vi "pf_Extract_Camera_Properties.vi"(8 "error in (no error)":errorcluster, 11 "IMAQ Session in":refnum<k11>) -> (0 "error out":errorcluster, 1 "Properties Array":T1[](array[typedef]), 3 "IMAQ Session out":refnum<k11>)   [LabVIEW 2025, in "Photonfocus_Toolkit.lvlib"]
uses:
  Photonfocus_Toolkit.lvlib
  _Private/Controls/pf_Property_Cluster.ctl
  _Private/Controls/pf_Property_Type.ctl
  _Private/Controls/pf_Property_Flag.ctl
  _Private/Controls/pf_Property_Info.ctl
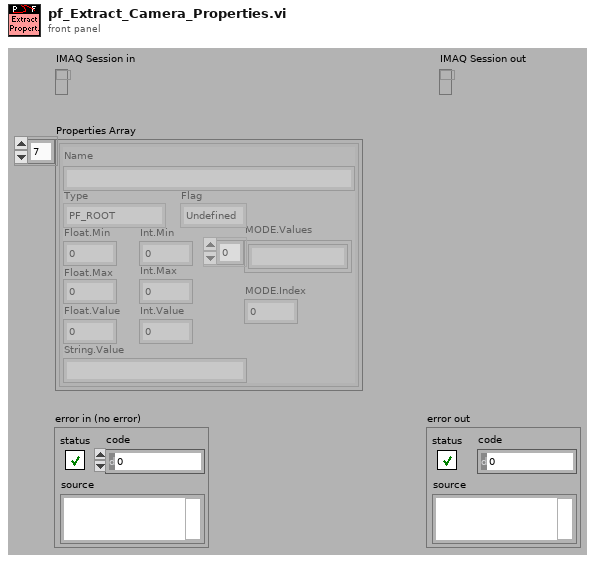
[diagram p1: front panel]
types:
  T1 = typedef "Photonfocus_Toolkit.lvlib/pf_Property_Cluster.ctl" = cluster{"Name":string, "Type":T2, "Float.Min":sgl, "Float.Max":sgl, "Float.Value":sgl, "Int.Min":u32, "Int.Max":u32, "Int.Value":u32, "String.Value":string, "MODE.Values":string[], "MODE.Index":i32, "Flag":T3}
  T2 = typedef "Photonfocus_Toolkit.lvlib/pf_Property_Type.ctl" = enum16{"Undefined", "PF_ROOT", "PF_INT", "PF_FLOAT", "PF_BOOL", "PF_MODE", "PF_REGISTER", "PF_STRING", "PF_BUFFER", "PF_STRUCT", "PF_ARRAY", "PF_COMMAND", "PF_EVENT"}
  T3 = typedef "Photonfocus_Toolkit.lvlib/pf_Property_Flag.ctl" = enum16{"Undefined", "RO", "WO", "RW"}
  T4 = typedef "Photonfocus_Toolkit.lvlib/pf_Property_Info.ctl" = cluster{"Name":string, "Type":T2, "Flag":T3}
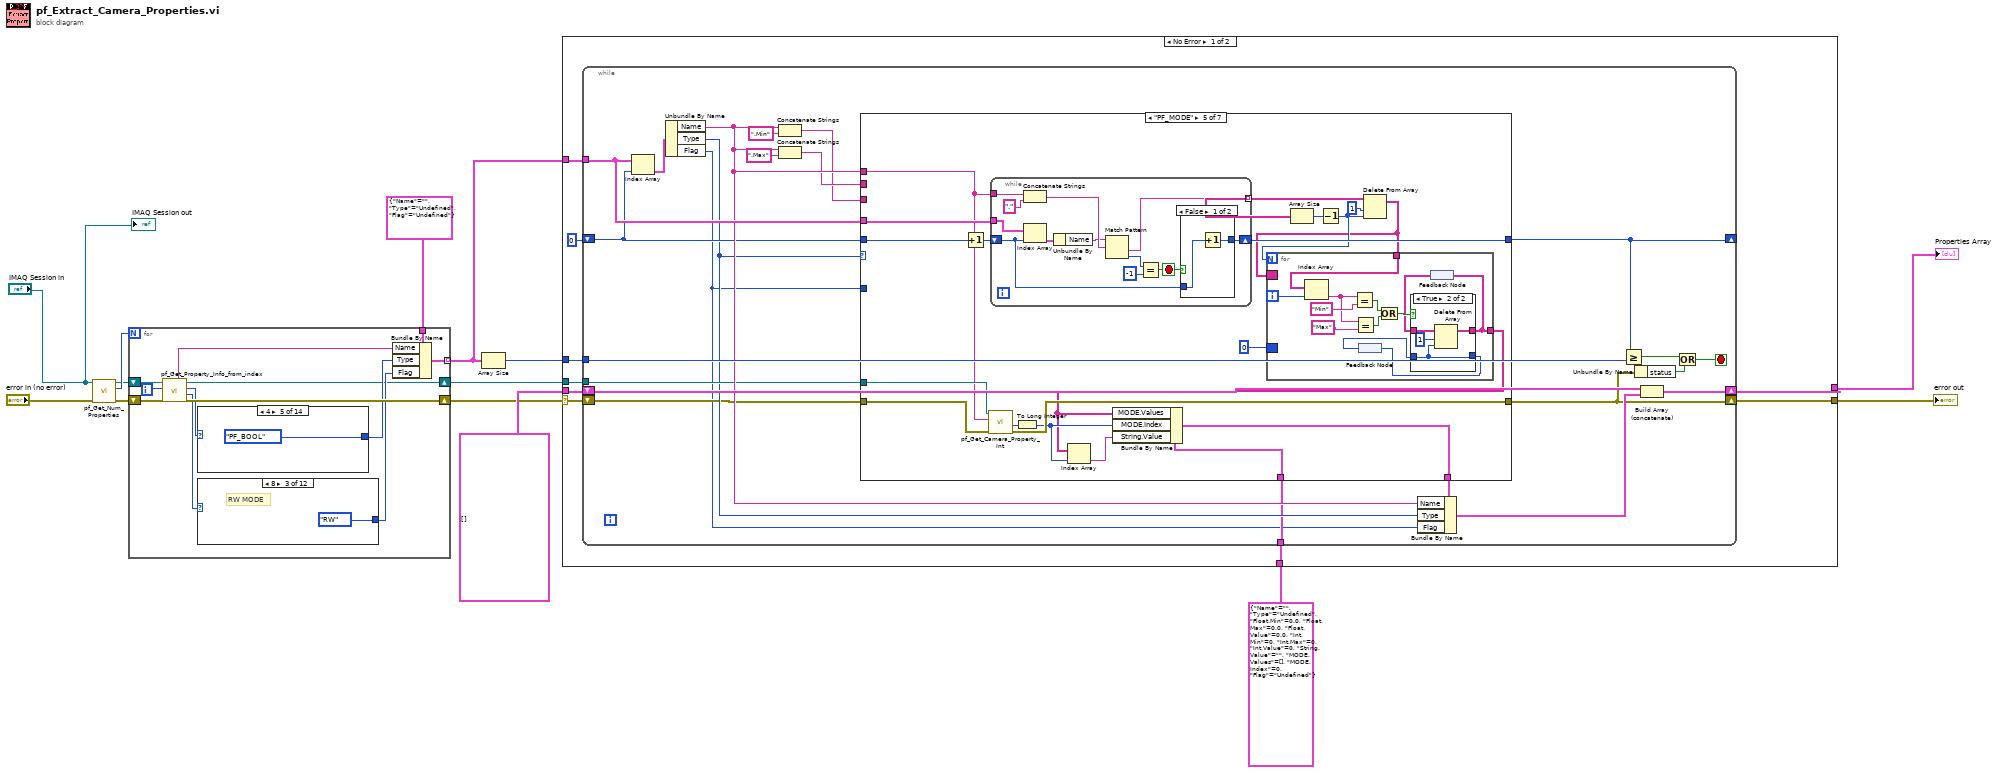
[diagram p0: block diagram]
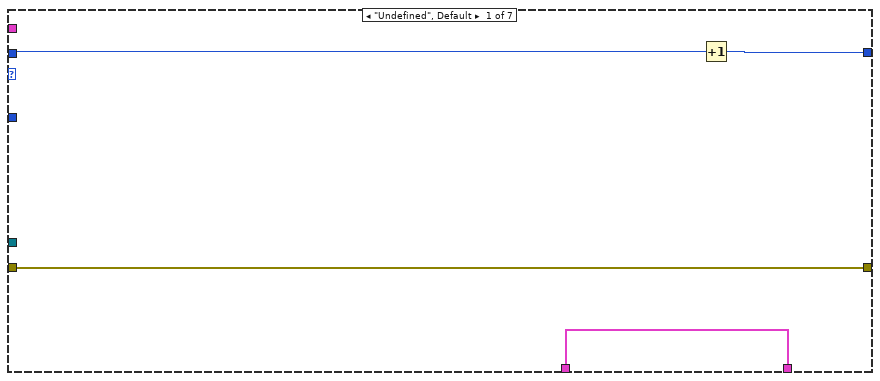
[diagram p2: hidden frame]
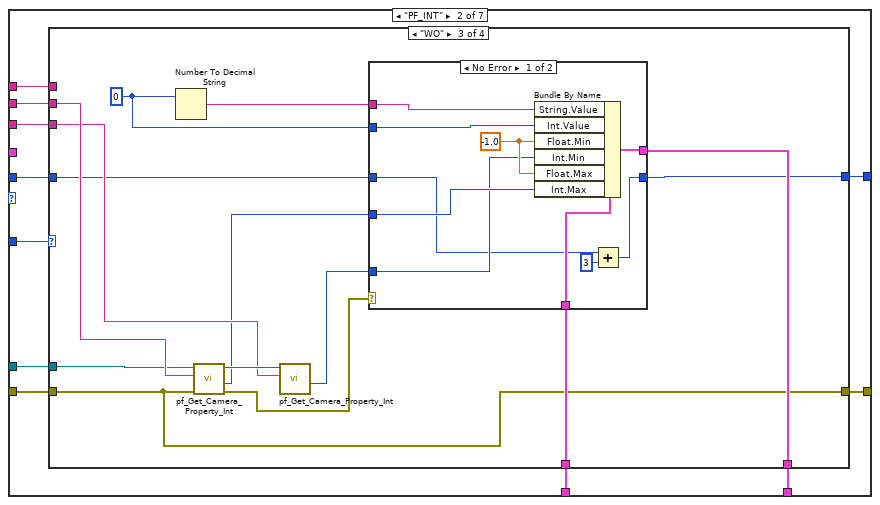
[diagram p3: hidden frame]
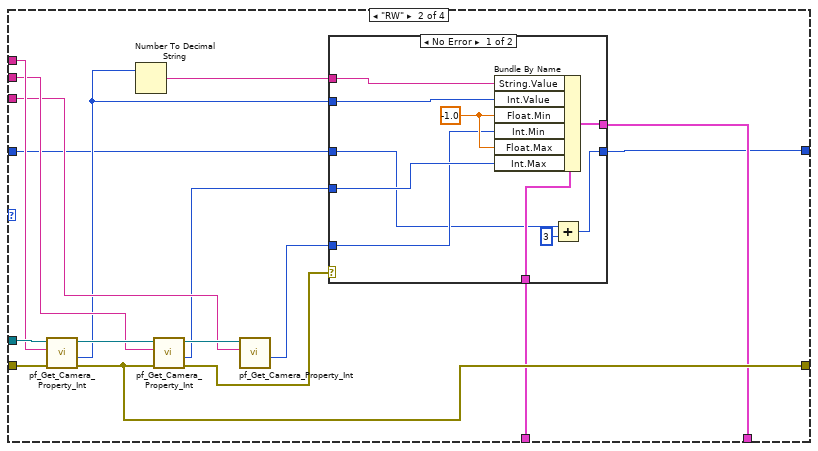
[diagram p5: hidden frame]
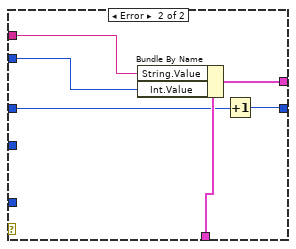
[diagram p6: hidden frame]
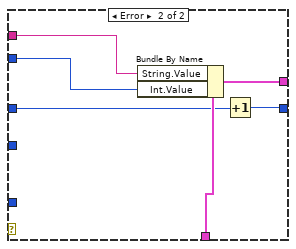
[diagram p7: hidden frame]
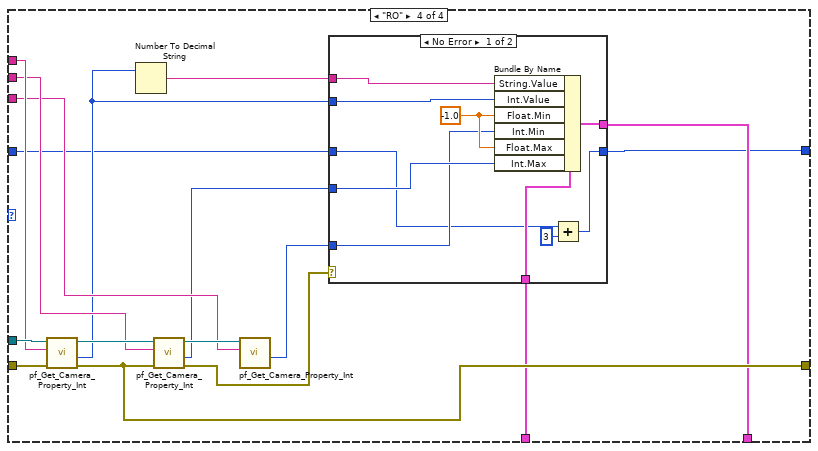
[diagram p8: hidden frame]
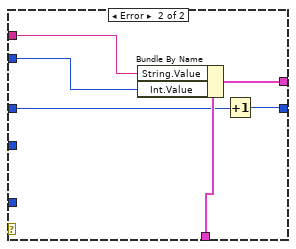
[diagram p9: hidden frame]
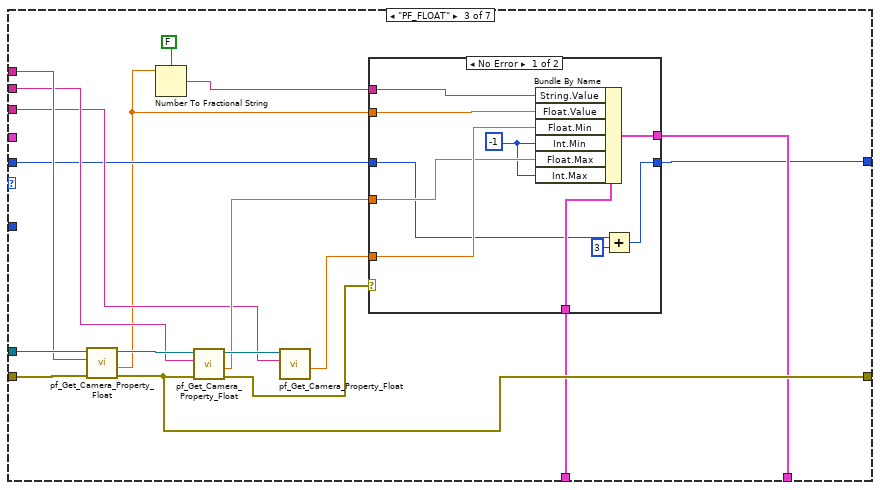
[diagram p10: hidden frame]
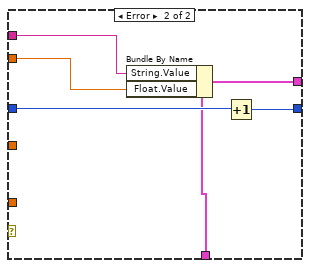
[diagram p11: hidden frame]
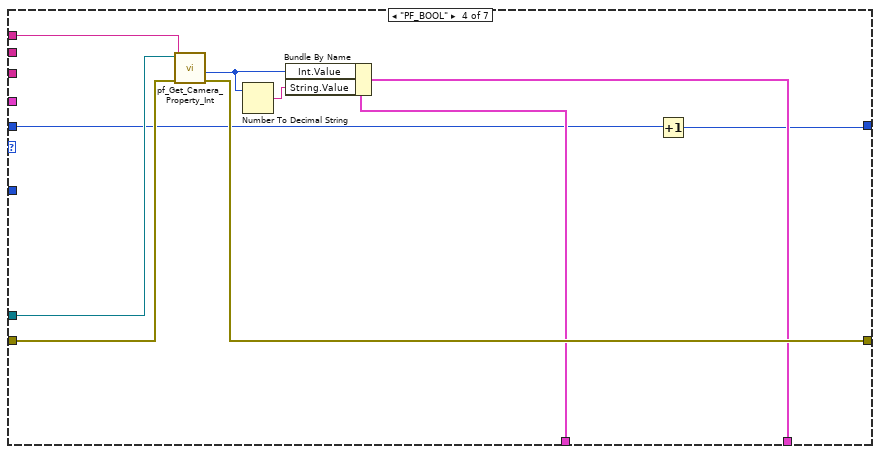
[diagram p12: hidden frame]
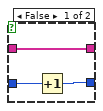
[diagram p13: hidden frame]
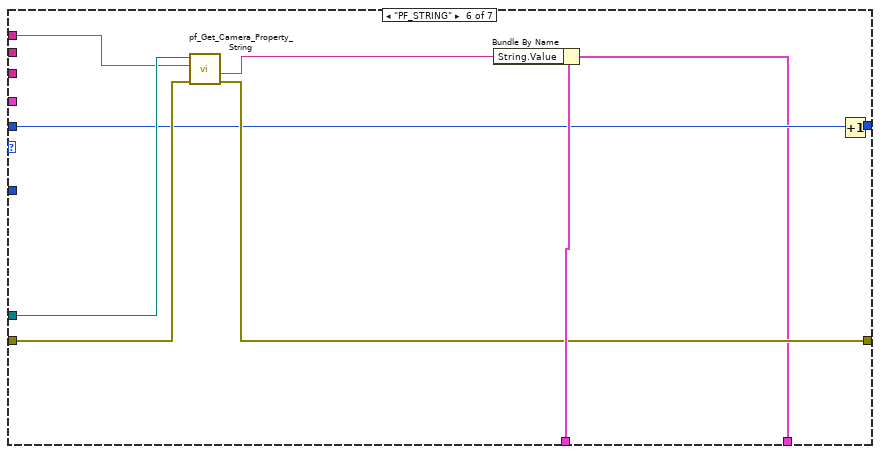
[diagram p15: hidden frame]
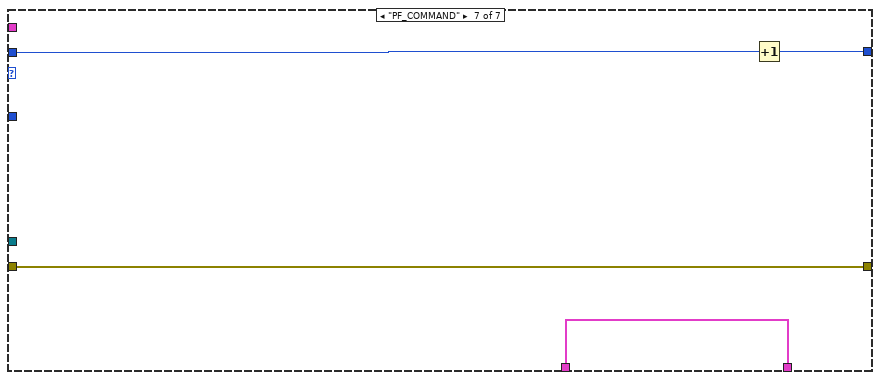
[diagram p16: hidden frame]
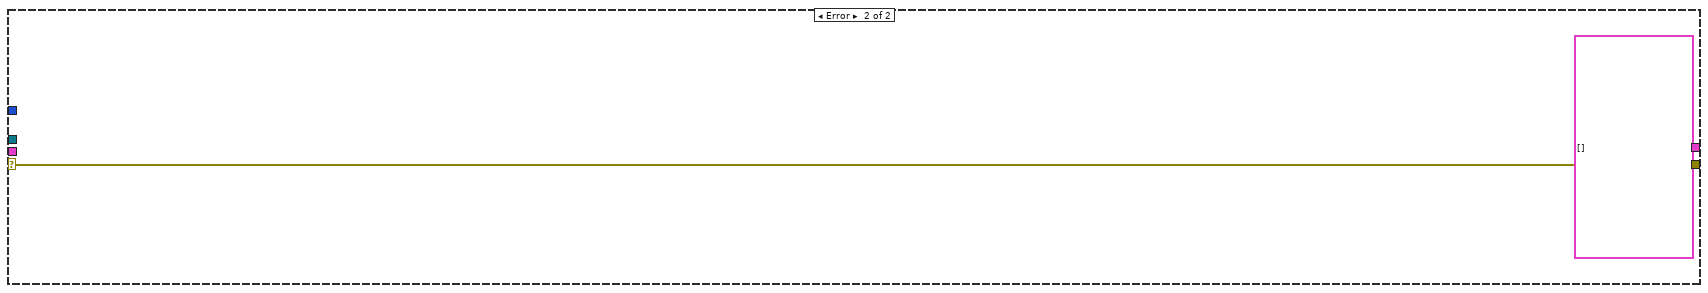
[diagram p17: hidden frame]
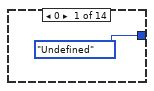
[diagram p18: hidden frame]
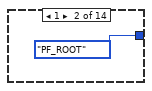
[diagram p19: hidden frame]
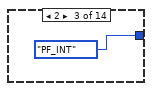
[diagram p20: hidden frame]
diagram:
  n1 = call "pf_Get_Num_Properties.vi"("error in (no error)"="error in (no error)", "IMAQ Session in"="IMAQ Session in") -> ("error out"=w12:errorcluster, "Number of Properties"=w5:i32, "IMAQ Session out"=w4:refnum<k11>)  [unwired: 7 out]
  n2 = for {
    N: w5 -> [_]
    shift-right: [w25] -> w8
    shift-left: w12 -> [w26]
    tunnel: T4 {"Name"="", "Type"=enum."Undefined", "Flag"=enum."Undefined"} ("Property Info 2") -> [w24]
    tunnel: [w23] -> w10 mode=indexing
    shift-right: [w15] -> w3
    shift-left: w4 -> [w17]
    i -> [w18]
    n3 = call "pf_Get_Property_Info_from_index.vi"("error in (no error)"=w26, "Property index"=w18, "IMAQ Session in"=w17) -> ("error out"=w25:errorcluster, "Property Flag"=w22:i32, "Property Type"=w19:i32, "IMAQ Session out"=w15:refnum<k11>, "Property Name"=w16:string)  [unwired: 4 out]
    n4 = case shown="4" w19 {
      tunnel: [pf_Property_Type."Undefined" ("Type") pf_Property_Type."PF_ROOT" ("Type") pf_Property_Type."PF_INT" ("Type") pf_Property_Type."PF_FLOAT" ("Type") pf_Property_Type."PF_BOOL" ("Type") pf_Property_Type."PF_MODE" ("Type") pf_Property_Type."PF_REGISTER" ("Type") pf_Property_Type."PF_STRING" ("Type") pf_Property_Type."PF_BUFFER" ("Type") pf_Property_Type."PF_STRUCT" ("Type") pf_Property_Type."PF_ARRAY" ("Type") pf_Property_Type."PF_COMMAND" ("Type") pf_Property_Type."PF_EVENT" ("Type") pf_Property_Type."Undefined" ("Type")] -> w20
      frame 0 {
      }
      frame 1 {
      }
      frame 2 {
      }
      frame 3 {
      }
      frame 4 {
      }
      frame 5 {
      }
      frame 6 {
      }
      frame 7 {
      }
      frame 8 {
      }
      frame 9 {
      }
      frame 10 {
      }
      frame 11 {
      }
      frame 12 {
      }
      frame Default {
      }
    }
    n5 = case shown="8" w22 {
      tunnel: [pf_Property_Flag."RW" ("Flag") pf_Property_Flag."Undefined" ("Flag") pf_Property_Flag."RW" ("Flag") pf_Property_Flag."RO" ("Flag") pf_Property_Flag."WO" ("Flag") pf_Property_Flag."WO" ("Flag") pf_Property_Flag."Undefined" ("Flag") pf_Property_Flag."Undefined" ("Flag") pf_Property_Flag."RW" ("Flag") pf_Property_Flag."RW" ("Flag") pf_Property_Flag."RO" ("Flag") pf_Property_Flag."Undefined" ("Flag")] -> w21
      frame 0 {
        # "RW MODE"
      }
      frame 4 {
      }
      frame 8 {
        # "RW MODE"
      }
      frame 16 {
        # "RO MODE ELEMENT"
      }
      frame 32 {
        # "WO COMMAND"
      }
      frame 40 {
        # "WO COMMAND"
      }
      frame 48 {
      }
      frame 56 {
      }
      frame 64 {
        # "PROPERTY IS CURRENTY INACTIVE"
      }
      frame 72 {
        # "RW FLOAT"
      }
      frame 80 {
        # "RO STRING"
      }
      frame Default {
      }
    }
    n6 = Bundle By Name(cluster=w24, "Name"=w16, "Type"=w20, "Flag"=w21) -> (w23:T4)
  }
  n7 = Array Size(array=w10) -> (size(s)=w14:i32)
  n8 = case shown="No Error" w8 {
    selector: w8 -> [w55 w311]
    tunnel: w14 -> [w60 _]
    tunnel: T1[] [] -> [w59 _]
    tunnel: w10 -> [w58 _]
    tunnel: [w57 T1[] []] -> w9
    tunnel: [w56 w311] -> w6
    tunnel: w3 -> [w54 _]
    tunnel: T1 {"Name"="", "Type"=enum."Undefined", "Float.Min"=0.0, "Float.Max"=0.0, "Float.Value"=0.0, "Int.Min"=0, "Int.Max"=0, "Int.Value"=0, "String.Value"="", "MODE.Values"=[], "MODE.Index"=0, "Flag"=enum."Undefined"} ("Cluster") -> [w53 _]
    frame No Error {
      n9 = while {
        tunnel: w58 -> [w74]
        shift-right: [w65] -> _
        shift-left: 0 -> [w71]
        tunnel: w60 -> [w84]
        shift-right: [w80] -> w57
        shift-left: w59 -> [w81]
        shift-right: [w66] -> w56
        shift-left: w55 -> [w69]
        tunnel: w54 -> [w72]
        tunnel: w53 -> [w68]
        stop <- w75 stop-if-true
        n10 = Index Array(array=w74, index=w71) -> (element=w79:T4)
        n11 = Unbundle By Name(w79) -> ("Name"=w73:string, "Type"=w70:T2, "Flag"=w62:T3)
        n12 = Concatenate Strings(w73, ".Min" ("string")) -> (w63:string)
        n13 = Concatenate Strings(w73, ".Max" ("string")) -> (w64:string)
        n14 = case shown="\"PF_MODE\"" w70 {
          tunnel: w68 -> [w87 w92 w205 w235 w262 w305 w308]
          tunnel: w73 -> [_ w97 w210 w238 w250 w301 _]
          tunnel: w74 -> [_ _ _ _ w261 _ _]
          tunnel: w71 -> [w86 w90 w207 w234 w260 w299 w307]
          tunnel: [w85 w91 w203 w233 w248 w298 w306] -> w65
          tunnel: w69 -> [w88 w99 w212 w242 w256 w304 w309]
          tunnel: [w88 w95 w206 w241 w255 w303 w309] -> w66
          tunnel: w72 -> [_ w98 w211 w239 w252 w302 _]
          tunnel: [w87 w93 w204 w236 w249 w297 w308] -> w67
          tunnel: w64 -> [_ w96 w209 _ _ _ _]
          tunnel: w63 -> [_ w94 w208 _ _ _ _]
          tunnel: w62 -> [_ w89 _ _ _ _ _]
          frame "Undefined", Default {
            n15 = Increment(x=w86) -> (x+1=w85:i32)
          }
          frame "PF_INT" {
            n16 = case shown="\"WO\"" w89 {
              tunnel: w99 -> [w102 w118 w137 w181]
              tunnel: w98 -> [_ w117 w136 w180]
              tunnel: w97 -> [_ w116 _ w179]
              tunnel: w96 -> [_ w115 w149 w178]
              tunnel: [w102 w113 w137 w176] -> w95
              tunnel: w94 -> [_ w112 w147 w175]
              tunnel: [w100 w107 w143 w170] -> w93
              tunnel: w92 -> [w100 w106 w142 w169]
              tunnel: [w101 w105 w141 w168] -> w91
              tunnel: w90 -> [w101 w104 w140 w167]
              frame "Undefined", Default {
              }
              frame "RW" {
                n17 = call "pf_Get_Camera_Property_Int.vi"("error in (no error)"=w118, "Property Name"=w116, "IMAQ Session in"=w117) -> ("error out"=w113:errorcluster, "Property Value"=w108:i32, "IMAQ Session out"=w119:refnum<k11>)  [unwired: 6 out]
                n18 = Number To Decimal String(number=w108) -> (decimal integer string=w109:string)  [unwired: 1 out]
                n19 = call "pf_Get_Camera_Property_Int.vi"("error in (no error)"=w113, "Property Name"=w115, "IMAQ Session in"=w119) -> ("error out"=w103:errorcluster, "Property Value"=w111:i32, "IMAQ Session out"=w114:refnum<k11>)  [unwired: 6 out]
                n20 = call "pf_Get_Camera_Property_Int.vi"("Property Name"=w112, "IMAQ Session in"=w114) -> ("Property Value"=w110:i32)  [unwired: 1 in, 8 out]
                n21 = case shown="No Error" w103 {
                  tunnel: w111 -> [w128 _]
                  tunnel: w110 -> [w127 _]
                  tunnel: w109 -> [w126 w133]
                  tunnel: w108 -> [w125 w132]
                  tunnel: [w124 w134] -> w107
                  tunnel: w106 -> [w123 w135]
                  tunnel: [w121 w130] -> w105
                  tunnel: w104 -> [w120 w131]
                  frame No Error {
                    w129 = -1.0 ("Value.F.min")
                    n22 = Bundle By Name(cluster=w123, "String.Value"=w126, "Int.Value"=w125, "Float.Min"=w129, "Int.Min"=w127, "Float.Max"=w129, "Int.Max"=w128) -> (w124:T1)
                    n23 = Add(x=w120, y=3) -> (x+y=w121:i32)
                  }
                  frame Error {
                    n24 = Bundle By Name(cluster=w135, "String.Value"=w133, "Int.Value"=w132) -> (w134:T1)
                    n25 = Increment(x=w131) -> (x+1=w130:i32)
                  }
                }
              }
              frame "WO" {
                w138 = 0 ("Value.I.max")
                n26 = Number To Decimal String(number=w138) -> (decimal integer string=w144:string)  [unwired: 1 out]
                n27 = call "pf_Get_Camera_Property_Int.vi"("error in (no error)"=w137, "Property Name"=w149, "IMAQ Session in"=w136) -> ("error out"=w139:errorcluster, "Property Value"=w146:i32, "IMAQ Session out"=w148:refnum<k11>)  [unwired: 6 out]
                n28 = call "pf_Get_Camera_Property_Int.vi"("Property Name"=w147, "IMAQ Session in"=w148) -> ("Property Value"=w145:i32)  [unwired: 1 in, 8 out]
                n29 = case shown="No Error" w139 {
                  tunnel: w146 -> [w158 _]
                  tunnel: w145 -> [w157 _]
                  tunnel: w144 -> [w156 w163]
                  tunnel: w138 -> [w155 w162]
                  tunnel: [w154 w164] -> w143
                  tunnel: w142 -> [w153 w165]
                  tunnel: [w151 w160] -> w141
                  tunnel: w140 -> [w150 w161]
                  frame No Error {
                    w159 = -1.0 ("Value.F.min")
                    n30 = Bundle By Name(cluster=w153, "String.Value"=w156, "Int.Value"=w155, "Float.Min"=w159, "Int.Min"=w157, "Float.Max"=w159, "Int.Max"=w158) -> (w154:T1)
                    n31 = Add(x=w150, y=3) -> (x+y=w151:i32)
                  }
                  frame Error {
                    n32 = Bundle By Name(cluster=w165, "String.Value"=w163, "Int.Value"=w162) -> (w164:T1)
                    n33 = Increment(x=w161) -> (x+1=w160:i32)
                  }
                }
              }
              frame "RO" {
                n34 = call "pf_Get_Camera_Property_Int.vi"("error in (no error)"=w181, "Property Name"=w179, "IMAQ Session in"=w180) -> ("error out"=w176:errorcluster, "Property Value"=w171:i32, "IMAQ Session out"=w182:refnum<k11>)  [unwired: 6 out]
                n35 = Number To Decimal String(number=w171) -> (decimal integer string=w172:string)  [unwired: 1 out]
                n36 = call "pf_Get_Camera_Property_Int.vi"("error in (no error)"=w176, "Property Name"=w178, "IMAQ Session in"=w182) -> ("error out"=w166:errorcluster, "Property Value"=w174:i32, "IMAQ Session out"=w177:refnum<k11>)  [unwired: 6 out]
                n37 = call "pf_Get_Camera_Property_Int.vi"("Property Name"=w175, "IMAQ Session in"=w177) -> ("Property Value"=w173:i32)  [unwired: 1 in, 8 out]
                n38 = case shown="No Error" w166 {
                  tunnel: w174 -> [w191 _]
                  tunnel: w173 -> [w190 _]
                  tunnel: w172 -> [w189 w196]
                  tunnel: w171 -> [w188 w195]
                  tunnel: [w187 w197] -> w170
                  tunnel: w169 -> [w186 w198]
                  tunnel: [w184 w193] -> w168
                  tunnel: w167 -> [w183 w194]
                  frame No Error {
                    w192 = -1.0 ("Value.F.min")
                    n39 = Bundle By Name(cluster=w186, "String.Value"=w189, "Int.Value"=w188, "Float.Min"=w192, "Int.Min"=w190, "Float.Max"=w192, "Int.Max"=w191) -> (w187:T1)
                    n40 = Add(x=w183, y=3) -> (x+y=w184:i32)
                  }
                  frame Error {
                    n41 = Bundle By Name(cluster=w198, "String.Value"=w196, "Int.Value"=w195) -> (w197:T1)
                    n42 = Increment(x=w194) -> (x+1=w193:i32)
                  }
                }
              }
            }
          }
          frame "PF_FLOAT" {
            n43 = call "pf_Get_Camera_Property_Float.vi"("error in (no error)"=w212, "Property Name"=w210, "IMAQ Session in"=w211) -> ("error out"=w206:errorcluster, "Property Value"=w201:sgl, "IMAQ Session out"=w216:refnum<k11>)  [unwired: 6 out]
            n44 = Number To Fractional String(use system decimal point (T)=FALSE, number=w201) -> (F-format string=w200:string)  [unwired: 2 out]
            n45 = call "pf_Get_Camera_Property_Float.vi"("error in (no error)"=w206, "Property Name"=w209, "IMAQ Session in"=w216) -> ("error out"=w199:errorcluster, "Property Value"=w214:sgl, "IMAQ Session out"=w215:refnum<k11>)  [unwired: 6 out]
            n46 = call "pf_Get_Camera_Property_Float.vi"("Property Name"=w208, "IMAQ Session in"=w215) -> ("Property Value"=w213:sgl)  [unwired: 1 in, 8 out]
            n47 = case shown="No Error" w199 {
              tunnel: w214 -> [w219 _]
              tunnel: w213 -> [w220 _]
              tunnel: w200 -> [w222 w228]
              tunnel: w201 -> [w221 w227]
              tunnel: [w224 w230] -> w204
              tunnel: w205 -> [w223 w229]
              tunnel: [w225 w231] -> w203
              tunnel: w207 -> [w217 w232]
              frame No Error {
                w218 = -1 ("Value.I.max")
                n48 = Bundle By Name(cluster=w223, "String.Value"=w222, "Float.Value"=w221, "Float.Min"=w220, "Int.Min"=w218, "Float.Max"=w219, "Int.Max"=w218) -> (w224:T1)
                n49 = Add(x=w217, y=3) -> (x+y=w225:i32)
              }
              frame Error {
                n50 = Bundle By Name(cluster=w229, "String.Value"=w228, "Float.Value"=w227) -> (w230:T1)
                n51 = Increment(x=w232) -> (x+1=w231:i32)
              }
            }
          }
          frame "PF_BOOL" {
            n52 = call "pf_Get_Camera_Property_Int.vi"("error in (no error)"=w242, "Property Name"=w238, "IMAQ Session in"=w239) -> ("error out"=w241:errorcluster, "Property Value"=w237:i32)  [unwired: 7 out]
            n53 = Number To Decimal String(number=w237) -> (decimal integer string=w240:string)  [unwired: 1 out]
            n54 = Bundle By Name(cluster=w235, "Int.Value"=w237, "String.Value"=w240) -> (w236:T1)
            n55 = Increment(x=w234) -> (x+1=w233:i32)
          }
          frame "PF_MODE" {
            n56 = Increment(x=w260) -> (x+1=w259:i32)
            n57 = call "pf_Get_Camera_Property_Int.vi"("error in (no error)"=w256, "Property Name"=w250, "IMAQ Session in"=w252) -> ("error out"=w255:errorcluster, "Property Value"=w251:i32)  [unwired: 7 out]
            n58 = while {
              shift-right: [w289] -> w248
              shift-left: w259 -> [w288]
              tunnel: w261 -> [w293]
              tunnel: w250 -> [w286]
              tunnel: [w287] -> w247 mode=indexing
              stop <- w290 stop-if-true
              n59 = Concatenate Strings(w286, "." ("string")) -> (w284:string)
              n60 = Index Array(array=w293, index=w288) -> (element=w283:T4)
              n61 = Unbundle By Name(w283) -> ("Name"=w282:string)
              n62 = Match Pattern(string=w282, regular expression=w284) -> (after substring=w287:string, offset past match=w292:i32)  [unwired: 3 out]
              n63 = Equal?(x=w292, y=-1) -> (x = y?=w290:bool)
              n64 = case shown="False" w290 {
                tunnel: [w295 w296] -> w289
                tunnel: w288 -> [w294 w296]
                frame False {
                  n65 = Increment(x=w294) -> (x+1=w295:i32)
                }
                frame True {
                }
              }
            }
            n66 = To Long Integer(number=w251) -> (32bit integer=w254:i32)
            n67 = Array Size(array=w247) -> (size(s)=w257:i32)
            n68 = Decrement(x=w257) -> (x-1=w245:i32)
            n69 = Delete From Array(array=w247, length=1, index=w245) -> (array with subset deleted=w243:string[])  [unwired: 1 out]
            n70 = for {
              N: w245 -> [_]
              tunnel: [w264] -> w246
              tunnel: w243 -> [w263]
              border: 0 ("length") -> [_]
              border: w243 -> [_]
              i -> [w268]
              n71 = Index Array(array=w263, index=w268) -> (element=w272:string)
              n72 = Equal?(x=w272, y="Min" ("string")) -> (x = y?=w270:bool)
              n73 = Equal?(x=w272, y="Max" ("string")) -> (x = y?=w271:bool)
              n74 = feedback #1() -> (w265:i32)
              n75 = Or(x=w270, y=w271) -> (x .or. y?=w269:bool)
              n76 = feedback #2() -> (w267:string[])
              n77 = case shown="True" w269 {
                tunnel: w267 -> [w277 w280]
                tunnel: [w277 w279] -> w264
                tunnel: [w276 w278] -> w266
                tunnel: w265 -> [w275 w278]
                frame False {
                  n78 = Increment(x=w275) -> (x+1=w276:i32)
                }
                frame True {
                  n79 = Delete From Array(array=w280, length=1, index=w278) -> (array with subset deleted=w279:string[])  [unwired: 1 out]
                }
              }
              n80 = feedback-in #1(w266) -> ()
              n81 = feedback-in #2(w264) -> ()
            }
            n82 = Index Array(array=w246, index=w254) -> (element=w253:string)
            n83 = Bundle By Name(cluster=w262, "MODE.Values"=w246, "MODE.Index"=w254, "String.Value"=w253) -> (w249:T1)
          }
          frame "PF_STRING" {
            n84 = call "pf_Get_Camera_Property_String.vi"("error in (no error)"=w304, "Property Name"=w301, "IMAQ Session in"=w302) -> ("error out"=w303:errorcluster, "String Value"=w300:string)  [unwired: 1 in, 6 out]
            n85 = Bundle By Name(cluster=w305, "String.Value"=w300) -> (w297:T1)
            n86 = Increment(x=w299) -> (x+1=w298:i32)
          }
          frame "PF_COMMAND" {
            n87 = Increment(x=w307) -> (x+1=w306:i32)
          }
        }
        n88 = Bundle By Name(cluster=w67, "Name"=w73, "Type"=w70, "Flag"=w62) -> (w78:T1)
        n89 = Greater Or Equal?(x=w65, y=w84) -> (x >= y?=w77:bool)
        n90 = Unbundle By Name(w66) -> ("status"=w76:bool)
        n91 = Build Array (concatenate)(w81, w78) -> (w80:T1[])
        n92 = Or(x=w77, y=w76) -> (x .or. y?=w75:bool)
      }
    }
    frame Error {
    }
  }
  "Properties Array" <- w9
  "error out" <- w6
  "IMAQ Session out" <- "IMAQ Session in"
